vi "V and A.vi"(7 "fps":dbl=10.0, 8 "total x (mm)":dbl=25.0) -> (3 "a":dbl, 5 "v2":dbl)   [LabVIEW 2022 SP3]
panel:
  out "t2":dbl
  out "t1":sgl
  out "x":dbl
  out "v1 don't use":dbl
  in  "velocity (ct/s)":dbl=10000.0 max=20000.0
  # "Maximum velocity 20 E6\n\nmax\nvelocity < (65536 × deceleration) – acceleration"
  # "Max acc is 2E9 with 125 microsecond sampling\nMax acc is 5E8 with 250 microsecond sampling"
  # "acc tune"
  # "constant V time"
  # "2t1+t2=1/fps"
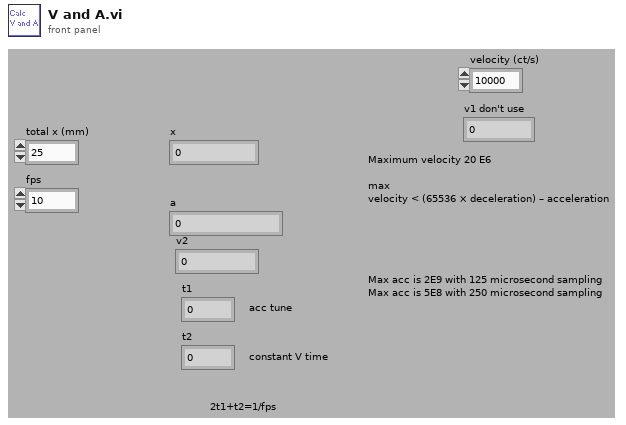
[diagram p1: front panel]
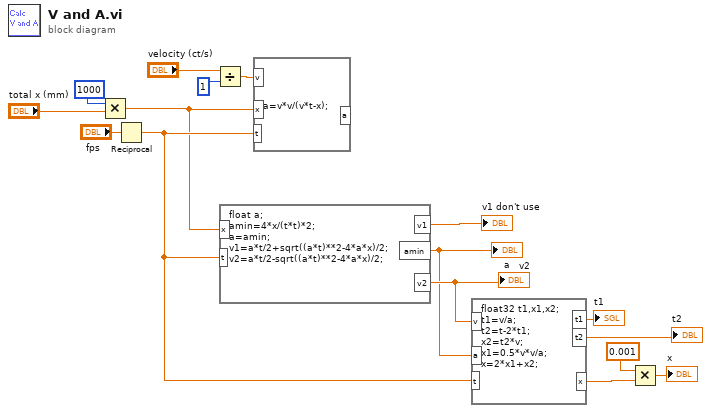
[diagram p0: block diagram]
diagram:
  n1 = Multiply(x=1000, y="total x (mm)") -> (x*y=w6:dbl)
  n2 = Reciprocal(x="fps") -> (1/x=w11:dbl)
  n3 = Divide(x="velocity (ct/s)", y=1) -> (x/y=w10:dbl)
  n4 = formula code="float a;\namin=4*x/(t*t)*2;\na=amin;\nv1=a*t/2+sqrt((a*t)**2-4*a*x)/2;\nv2=a*t/2-sqrt((a*t)**2-4*a*x)/2;"("x"=w6, "t"=w11) -> ("v1"=→"v1 don't use":dbl, "v2"=w2:dbl, "amin"=w1:dbl)
  "v2" <- w2
  "a" <- w1
  n5 = formula code="a=v*v/(v*t-x);"("v"=w10, "x"=w6, "t"=w11) -> ()  [unwired: 1 out]
  n6 = formula code="float32 t1,x1,x2;\nt1=v/a;\nt2=t-2*t1;\nx2=t2*v;\nx1=0.5*v*v/a;\nx=2*x1+x2;"("a"=w1, "v"=w2, "t"=w11) -> ("x"=w5:dbl, "t1"=→"t1":sgl, "t2"=→"t2":dbl)
  n7 = Multiply(x=0.001, y=w5) -> (x*y=→"x":dbl)
